vi "Initialize.vi"(8 "error in":errorcluster, 11 "Plugin in":refnum<class "Statistic.lvclass">) -> (0 "error out":errorcluster, 3 "Plugin out":refnum<class "Statistic.lvclass">)   [LabVIEW 2025, in "Statistic.lvlib" / "Statistic.lvclass"]
uses:
  Statistic.lvclass
  C:/Program Files/National Instruments/LabVIEW 2025/vi.lib/FlexLogger/SDK/PluginSDK.lvlibp/PEFClasses/SDK/Plugin/Plugin.lvclass
  <vilib>/FlexLogger/SDK/PluginSDK.lvlibp/PEFClasses/SDK/Processing Element/Timing Parameters.ctl
  <vilib>/FlexLogger/SDK/PluginSDK.lvlibp/PEFClasses/SDK/Processing Element/Timing Method.ctl
  Statistic.lvclass/Statistic.ctl
  <vilib>/FlexLogger/SDK/PluginSDK.lvlibp/PEFClasses/SDK/Plugin/ParameterAccess/Write DBL.vi
  <vilib>/FlexLogger/SDK/PluginSDK.lvlibp/PEFClasses/SDK/Plugin/ParameterAccess/Write Boolean.vi
  <vilib>/FlexLogger/SDK/PluginSDK.lvlibp/PEFClasses/SDK/Plugin/ParameterAccess/Write N Channel.vi
  <vilib>/FlexLogger/SDK/PluginSDK.lvlibp/PEFClasses/SDK/Plugin/Plugin.lvclass
  C:/Program Files/National Instruments/LabVIEW 2025/vi.lib/FlexLogger/SDK/PluginSDK.lvlibp/PEFClasses/SDK/Processing Element/Processing Element.lvclass
  C:/Users/Tester/Documents/LabVIEW Projects/FlexLogger IO Plug-ins/Statistic/Statistic.lvclass
  <vilib>/FlexLogger/SDK/PluginSDK.lvlibp/PEFClasses/SDK/Processing Element/Processing Element.lvclass
  kernel32.dll
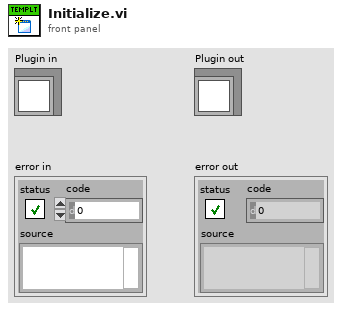
[diagram p1: front panel]
types:
  T1 = typedef "PluginSDK.lvlibp/Processing Element.lvclass/Timing Parameters.ctl" = cluster{"Timing Method":T2, "Timing Period (ms)":i32}
  T2 = typedef "PluginSDK.lvlibp/Processing Element.lvclass/Timing Method.ctl" = enum16{"Periodic", "Immediate", "On Data Ready", "Triggered"}
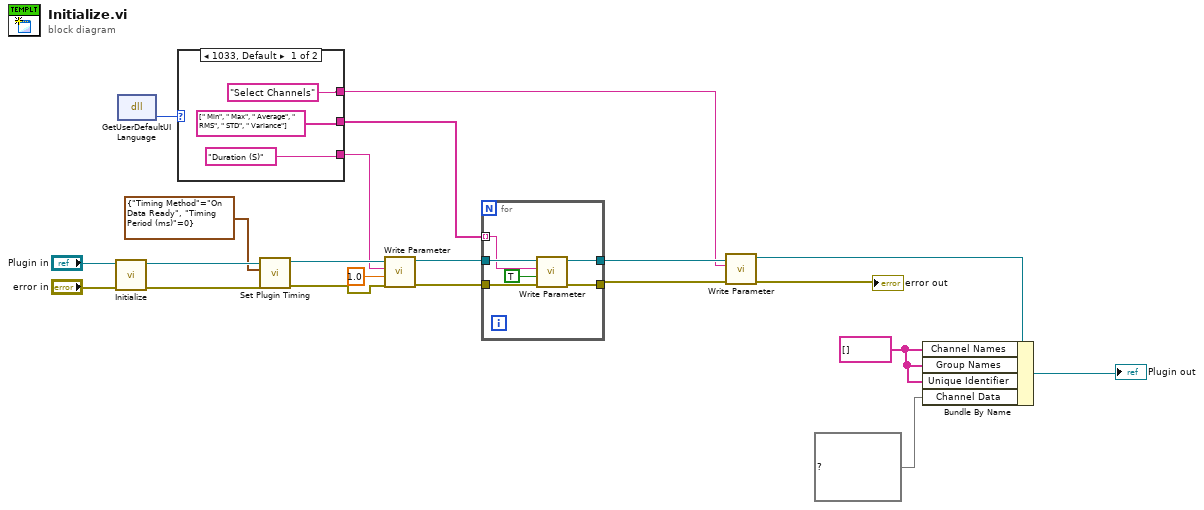
[diagram p0: block diagram]
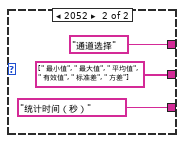
[diagram p2: hidden frame]
diagram:
  w19 = string[] [] ("Channel Names")
  n1 = call-parent "Initialize.vi"("error in (no error)"="error in", "Plugin in"="Plugin in") -> ("error out"=w8:errorcluster, "Plugin out"=w9:refnum<class "Statistic.lvclass">)  [unwired: 8 in]
  n2 = dll-call lib="kernel32.dll" fn="GetUserDefaultUILanguage"() -> ("return type"=w6:u16)  [unwired: 3 in, 2 out]
  n3 = case shown="1033, Default" w6 {
    tunnel: ["Select Channels" ("Name") "通道选择" ("Name")] -> w5
    tunnel: [string[] [" Min", " Max", " Average", " RMS", " STD", " Variance"] ("Unique Identifier") string[] [" 最小值", " 最大值", " 平均值", " 有效值", " 标准差", " 方差"] ("Unique Identifier")] -> w4
    tunnel: ["Duration (S)" ("Name") "统计时间（秒）" ("Name")] -> w3
    frame 1033, Default {
    }
    frame 2052 {
    }
  }
  n4 = call <vilib>:"Set Plugin Timing.vi"("error in (no error)"=w8, "Timing Parameters"=T1 {"Timing Method"=enum."On Data Ready", "Timing Period (ms)"=0}, "Plugin in"=w9) -> ("error out"=w14:errorcluster, "Plugin out"=w15:refnum<class "Statistic.lvclass">)  [unwired: 7 in]
  n5 = call-poly <vilib>:"Write Parameter.vi"("error in (no error)"=w14, "Value"=1.0, "Name"=w3, "Plugin in"=w15) -> ("error out"=w16:errorcluster, "Plugin out"=w17:refnum<class "Statistic.lvclass">)  [unwired: 6 in]
  n6 = for {
    tunnel: w17 -> [w33]
    tunnel: [w32] -> w12
    tunnel: w16 -> [w31]
    tunnel: [w30] -> w11
    tunnel: w4 -> [w29] mode=indexing
    n7 = call-poly <vilib>:"Write Parameter.vi"("error in (no error)"=w31, "Value"=TRUE, "Name"=w29, "Plugin in"=w33) -> ("error out"=w30:errorcluster, "Plugin out"=w32:refnum<class "Statistic.lvclass">)  [unwired: 6 in]
  }
  n8 = call-poly <vilib>:"Write Parameter.vi"("error in (no error)"=w11, "Name (Unique Channel Identifier)"=w5, "Plugin in"=w12) -> ("error out"=→"error out":errorcluster, "Plugin out"=w10:refnum<class "Statistic.lvclass">)  [unwired: 7 in]
  n9 = Bundle By Name(cluster=w10, "Channel Names"=w19, "Group Names"=w19, "Unique Identifier"=w19, "Channel Data"=map{string, dbl[]} {}) -> (→"Plugin out":refnum<class "Statistic.lvclass">)
